vi "saveparams.vi"(1 "timestamp":timestamp, 2 "filename prefix in":string, 3 "data dir in":path=path "C:/Users/Labmember/Desktop/Data/temp" caption="data dir.") -> ()   [LabVIEW 2015]
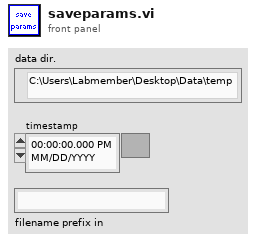
[diagram p1: front panel]
types:
  T1 = typedef "LVRectTypeDef.ctl" = cluster{"Left":i16, "Top":i16, "Right":i16, "Bottom":i16}
  T2 = cluster{"Xpixels":i32, "Vxminref":dbl, "Vxmaxref":dbl, "P":dbl, "Ypixels":i32, "Vyminref":dbl, "Vymaxref":dbl, "srate":sgl, "sAOxy":i32, "timeout":dbl, "type":string, "date":string, "time":string, "Colormap":u16, "Drawing Mode":u16, "Scanning Mode":u16, "square pixels":bool, "square matrix":bool, "Xpixels Img":i32, "Vx-min Img":dbl, "VX-max Img":dbl, "Ypixels Img":i32, "Vy-min Img":dbl, "Vy-max Img ":dbl, "Angle Img":dbl, "autoshutter":bool, "finite":bool, "cont":bool, "wavdet":bool, "measpoints":i32, "avpp":i32, "bufferAO":i32, "bufferAI":i32, "starttick":u32, "waveform":path, "Vx-ref":dbl, "Vy-ref":dbl, "refreshrate":dbl, "refreshbuffer":i32, "tt_cycles":i32, "motorref":refnum<k7>, "mirrorswitch":refnum<k7>, "sample mode":i32, "maxbufferAI":i32, "srateAODO":sgl, "bin":sgl, "Pel":sgl, "Angle draw":dbl, "srate Img":sgl, "ROIimg_plotbounds":T1, "auto OD":bool, "ODfilt":u16, "aAI":i32[], "aCI":i32[], "aAO":u32[], "aDO":u32[], "refwfsize":dbl, "Lifetime":bool, "Vz-Img":dbl, "Vz-ref":dbl, "Vz-reset":dbl, "AIoverride":bool}
  T3 = cluster{"VC":bool, "CC":bool, "CC_icg (pA/mv)":sgl, "VC_icg (mV/mV)":sgl, "OCG (mV/pA)":sgl, "OVG (mV/mV)":dbl, "Vhold (mV)":sgl, "holdon":bool}
  T4 = cluster{"initialized":bool, "devidx":i32, "Ch0 Level":i32, "Ch0 ZeroX":i32, "Ch1 Level":i32, "Ch1 ZeroX":i32, "sync rate":i32, "resolution":i32, "acq time":i32, "acq rate":i32, "# bins":u32, "Bin size":enum16{"1", "2", "4", "8", "16", "32", "64", "128"}, "min photons":u32, "truncate":u32}
  T5 = typedef "XYZStage.lvlib/XYZStage Configuration.ctl" = cluster{"VISA resource name":refnum<visa-resource-name>, "Timeout (3sec)":u32}
  T6 = cluster{"StageS":i32, "StageL":i32, "currmeas data dir":path, "image OD":u16, "contour OD":u16, "point OD":u16, "AOlines":tag[], "AIlines":tag[], "CI lines":tag[], "DO lines":tag[], "AO names":string[], "CI names":string[], "AI names":string[], "DO names":string[], "CIextensions":string[], "AIextensions":string[], "Voltage to Ygalvo":i32, "Voltage to Xgalvo":i32, "Voltage to patch":i32, "640 shutter":i32, "2P shutter":i32, "LT timestamp":u32, "Vp":i32, "Ip":i32, "camera trigger":i32, "master data dir":path, "voltage to Zpos":i32, "Vto2P":i32, "640 AO":i32, "488 AO":i32, "532 AO":i32, "640TTL":u32, "488TTL":u32, "532TTL":u32, "Device 1 sampleclock out":tag, "Device 1 Starttrigger out":tag, "Device 2 sampleclock in":tag, "Device 2 StartTrigger in ":tag, "2PODTTL":u32, "488 shutter":u32, "LCVR red":u32, "LCVR blue":u32, "Sutter Stage Config":T5}
  T7 = cluster{"AO parameters":cluster{"AOtab":dbl, "Repeats":dbl, "Cycles":dbl, "Start amplitude (V)":dbl, "Baseline (V)":dbl, "Step size (V)":dbl, "DC (%)":dbl, "Sampling frequency (Hz)":dbl, "Period (ms)":dbl, "Offset (V)":dbl, "Amplitude (V)":dbl, "Frequency":dbl, "Tri Repeats":dbl, "phase shift (ms)":dbl, "Pulses":dbl, "Matlab wave file":path, "Tri phase":dbl, "padding value":dbl}[], "DO parameters":cluster{"Digital DC (%)":dbl, "Digital phase":dbl, "Digital Freq (Hz)":dbl, "Sampling frequency (Hz)":dbl, "Digital time offset (s) ":dbl, "padding value":dbl, "matlab wave file":path, "DOtab":dbl}[]}
  T8 = cluster{"used AO lines":tag[], "used AO names":string[]}
  T9 = cluster{"used DO lines":tag[], "used DO names":string[]}
  T10 = cluster{"params out":cluster{"Xpixels":i32, "Vxminref":dbl, "Vxmaxref":dbl, "P":dbl, "Ypixels":i32, "Vyminref":dbl, "Vymaxref":dbl, "srate":sgl, "sAOxy":i32, "timeout":dbl, "type":string, "date":string, "time":string, "Colormap":u16, "Drawing Mode":u16, "Scanning Mode":u16, "square pixels":bool, "square matrix":bool, "Xpixels Img":i32, "Vx-min Img":dbl, "VX-max Img":dbl, "Ypixels Img":i32, "Vy-min Img":dbl, "Vy-max Img ":dbl, "Angle Img":dbl, "autoshutter":bool, "finite":bool, "cont":bool, "wavdet":bool, "measpoints":i32, "avpp":i32, "bufferAO":i32, "bufferAI":i32, "starttick":u32, "waveform":path, "Vx-ref":dbl, "Vy-ref":dbl, "refreshrate":dbl, "refreshbuffer":i32, "tt_cycles":i32, "motorref":refnum<k7>, "mirrorswitch":refnum<k7>, "sample mode":i32, "maxbufferAI":i32, "srateAODO":sgl, "bin":sgl, "Pel":sgl, "Angle draw":dbl, "srate Img":sgl, "ROIimg_plotbounds":T1, "auto OD":bool, "ODfilt":u16, "aAI":i32[], "aCI":i32[], "aAO":u32[], "aDO":u32[], "refwfsize":dbl, "Lifetime":bool, "Vz-Img":dbl, "Vz-ref":dbl, "Vz-reset":dbl, "AIoverride":bool}, "Params out":cluster{"VC":bool, "CC":bool, "CC_icg (pA/mv)":sgl, "VC_icg (mV/mV)":sgl, "OCG (mV/pA)":sgl, "OVG (mV/mV)":dbl, "Vhold (mV)":sgl, "holdon":bool}, "Params out":cluster{"initialized":bool, "devidx":i32, "Ch0 Level":i32, "Ch0 ZeroX":i32, "Ch1 Level":i32, "Ch1 ZeroX":i32, "sync rate":i32, "resolution":i32, "acq time":i32, "acq rate":i32, "# bins":u32, "Bin size":enum16{"1", "2", "4", "8", "16", "32", "64", "128"}, "min photons":u32, "truncate":u32}, "config out":cluster{"StageS":i32, "StageL":i32, "currmeas data dir":path, "image OD":u16, "contour OD":u16, "point OD":u16, "AOlines":tag[], "AIlines":tag[], "CI lines":tag[], "DO lines":tag[], "AO names":string[], "CI names":string[], "AI names":string[], "DO names":string[], "CIextensions":string[], "AIextensions":string[], "Voltage to Ygalvo":i32, "Voltage to Xgalvo":i32, "Voltage to patch":i32, "640 shutter":i32, "2P shutter":i32, "LT timestamp":u32, "Vp":i32, "Ip":i32, "camera trigger":i32, "master data dir":path, "voltage to Zpos":i32, "Vto2P":i32, "640 AO":i32, "488 AO":i32, "532 AO":i32, "640TTL":u32, "488TTL":u32, "532TTL":u32, "Device 1 sampleclock out":tag, "Device 1 Starttrigger out":tag, "Device 2 sampleclock in":tag, "Device 2 StartTrigger in ":tag, "2PODTTL":u32, "488 shutter":u32, "LCVR red":u32, "LCVR blue":u32, "Sutter Stage Config":T5}, "Params out":cluster{"AO parameters":cluster{"AOtab":dbl, "Repeats":dbl, "Cycles":dbl, "Start amplitude (V)":dbl, "Baseline (V)":dbl, "Step size (V)":dbl, "DC (%)":dbl, "Sampling frequency (Hz)":dbl, "Period (ms)":dbl, "Offset (V)":dbl, "Amplitude (V)":dbl, "Frequency":dbl, "Tri Repeats":dbl, "phase shift (ms)":dbl, "Pulses":dbl, "Matlab wave file":path, "Tri phase":dbl, "padding value":dbl}[], "DO parameters":cluster{"Digital DC (%)":dbl, "Digital phase":dbl, "Digital Freq (Hz)":dbl, "Sampling frequency (Hz)":dbl, "Digital time offset (s) ":dbl, "padding value":dbl, "matlab wave file":path, "DOtab":dbl}[]}, cluster{"used AO lines":tag[], "used AO names":string[]}, cluster{"used DO lines":tag[], "used DO names":string[]}}
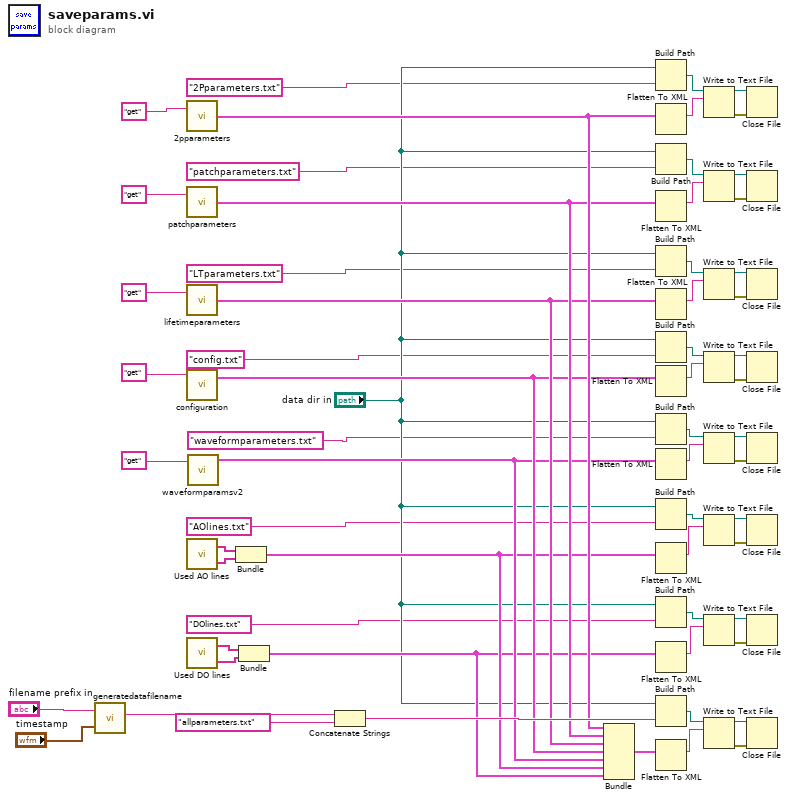
[diagram p0: block diagram]
diagram:
  n1 = call "generatedatafilename.vi"("timestamp"="timestamp", "filename prefix in"="filename prefix in") -> ("full-filename"=w15:string)
  n2 = call "2pparameters.vi"("command"="get") -> ("params out"=w49:T2)  [unwired: 1 in]
  n3 = call "patchparameters.vi"("command"="get") -> ("Params out"=w44:T3)  [unwired: 1 in]
  n4 = call "lifetimeparameters.vi"("command"="get") -> ("Params out"=w39:T4)  [unwired: 1 in]
  n5 = call "configuration.vi"("command"="get") -> ("config out"=w34:T6)  [unwired: 2 in, 1 out]
  n6 = call "Used AO lines.vi"() -> ("used AO names"=w27:string[], "used AO lines"=w28:tag[])  [unwired: 2 in]
  n7 = call "Used DO lines.vi"() -> ("used DO names"=w25:string[], "used DO lines"=w26:tag[])  [unwired: 2 in]
  n8 = call "waveformparamsv2.vi"("command"="get") -> ("Params out"=w29:T7)  [unwired: 4 in, 2 out]
  n9 = Bundle("used AO lines"=w28, "used AO names"=w27) -> (w20:T8)  [unwired: 1 in]
  n10 = Bundle("used DO lines"=w26, "used DO names"=w25) -> (w14:T9)  [unwired: 1 in]
  n11 = Concatenate Strings(w15, "allparameters.txt" ("string")) -> (w61:string)
  n12 = Bundle("params out"=w49, "Params out"=w44, "Params out"=w39, "config out"=w34, "Params out"=w29, w20, w14) -> (w57:T10)  [unwired: 1 in]
  n13 = Build Path(base path="data dir in", name or relative path="2Pparameters.txt" ("string")) -> (appended path=w50:path)
  n14 = Flatten To XML(anything=w49) -> (xml string=w53:string)
  n15 = Build Path(base path="data dir in", name or relative path="patchparameters.txt" ("string")) -> (appended path=w48:path)
  n16 = Flatten To XML(anything=w44) -> (xml string=w45:string)
  n17 = Build Path(base path="data dir in", name or relative path="LTparameters.txt" ("string")) -> (appended path=w40:path)
  n18 = Flatten To XML(anything=w39) -> (xml string=w43:string)
  n19 = Build Path(base path="data dir in", name or relative path="config.txt" ("string")) -> (appended path=w38:path)
  n20 = Flatten To XML(anything=w34) -> (xml string=w35:string)
  n21 = Build Path(base path="data dir in", name or relative path="waveformparameters.txt" ("string")) -> (appended path=w30:path)
  n22 = Flatten To XML(anything=w29) -> (xml string=w33:string)
  n23 = Build Path(base path="data dir in", name or relative path="AOlines.txt" ("string")) -> (appended path=w24:path)
  n24 = Flatten To XML(anything=w20) -> (xml string=w21:string)
  n25 = Build Path(base path="data dir in", name or relative path="DOlines.txt" ("string")) -> (appended path=w16:path)
  n26 = Flatten To XML(anything=w14) -> (xml string=w19:string)
  n27 = Build Path(base path="data dir in", name or relative path=w61) -> (appended path=w58:path)
  n28 = Flatten To XML(anything=w57) -> (xml string=w56:string)
  n29 = Write to Text File(file (use dialog)=w50, text=w53) -> (refnum out=w51:refnum<file>, error out=w52:errorcluster)  [unwired: 2 in, 1 out]
  n30 = Write to Text File(file (use dialog)=w48, text=w45) -> (refnum out=w47:refnum<file>, error out=w46:errorcluster)  [unwired: 2 in, 1 out]
  n31 = Write to Text File(file (use dialog)=w40, text=w43) -> (refnum out=w41:refnum<file>, error out=w42:errorcluster)  [unwired: 2 in, 1 out]
  n32 = Write to Text File(file (use dialog)=w38, text=w35) -> (refnum out=w37:refnum<file>, error out=w36:errorcluster)  [unwired: 2 in, 1 out]
  n33 = Write to Text File(file (use dialog)=w30, text=w33) -> (refnum out=w31:refnum<file>, error out=w32:errorcluster)  [unwired: 2 in, 1 out]
  n34 = Write to Text File(file (use dialog)=w24, text=w21) -> (refnum out=w23:refnum<file>, error out=w22:errorcluster)  [unwired: 2 in, 1 out]
  n35 = Write to Text File(file (use dialog)=w16, text=w19) -> (refnum out=w17:refnum<file>, error out=w18:errorcluster)  [unwired: 2 in, 1 out]
  n36 = Write to Text File(file (use dialog)=w58, text=w56) -> (refnum out=w60:refnum<file>, error out=w59:errorcluster)  [unwired: 2 in, 1 out]
  n37 = Close File(refnum=w51, error in=w52) -> ()  [unwired: 2 out]
  n38 = Close File(refnum=w47, error in=w46) -> ()  [unwired: 2 out]
  n39 = Close File(refnum=w41, error in=w42) -> ()  [unwired: 2 out]
  n40 = Close File(refnum=w37, error in=w36) -> ()  [unwired: 2 out]
  n41 = Close File(refnum=w31, error in=w32) -> ()  [unwired: 2 out]
  n42 = Close File(refnum=w23, error in=w22) -> ()  [unwired: 2 out]
  n43 = Close File(refnum=w17, error in=w18) -> ()  [unwired: 2 out]
  n44 = Close File(refnum=w60, error in=w59) -> ()  [unwired: 2 out]
